vi "test-trapezoid-profile-switch-goal-in-middle-2.vi"() -> ()   [LabVIEW 2019]
uses:
  <vilib>/Rock Robotics/WPI/ThirdParty/JAS_Junk/TrajLib/TRAPEZOID_PROFILE_STATE.ctl
  <vilib>/Rock Robotics/WPI/ThirdParty/JAS_Junk/TrajLib/TRAPEZOID_PROFILE.ctl
  <vilib>/Rock Robotics/WPI/ThirdParty/JAS_Junk/TrajLib/TRAPEZOID_PROFILE_CONSTRAINT.ctl
  <vilib>/Rock Robotics/WPI/ThirdParty/JAS_Junk/TrajLib/TrapProfile_ShouldFlipAcceleration.vi
  <vilib>/Rock Robotics/WPI/ThirdParty/JAS_Junk/TrajLib/TrapProfile_Direct.vi
  <vilib>/Rock Robotics/SystemInterfaces/NetworkCommunication/NetComm_UsageReport_report.vi
  <vilib>/Rock Robotics/WPI/ThirdParty/JAS_Junk/TrajLib/Util_LibraryGlobals.vi
  <vilib>/Rock Robotics/WPI/ThirdParty/JAS_Junk/TrajLib/Trajectory_Library.lvlib
panel:
  out "TRAPEZOID_PROFILE":T1 {"Goal"."Velocity" format="%16_6e"; "Goal"."Position" format="%16_6e"; "Initial"."Velocity" format="%16_6e"; "Initial"."Position" format="%16_6e"; "Constraints"."MaxAcceleration" format="%16_6e"; "Constraints"."MaxVelocity" format="%16_6e"; "EndDecel" format="%16_6e"; "EndFullSpeed" format="%16_6e"; "EndAccel" format="%16_6e"}
  out "State":T3 {"Velocity" format="%16_6e"; "Position" format="%16_6e"}
  out "Waveform Chart":T4(graph)
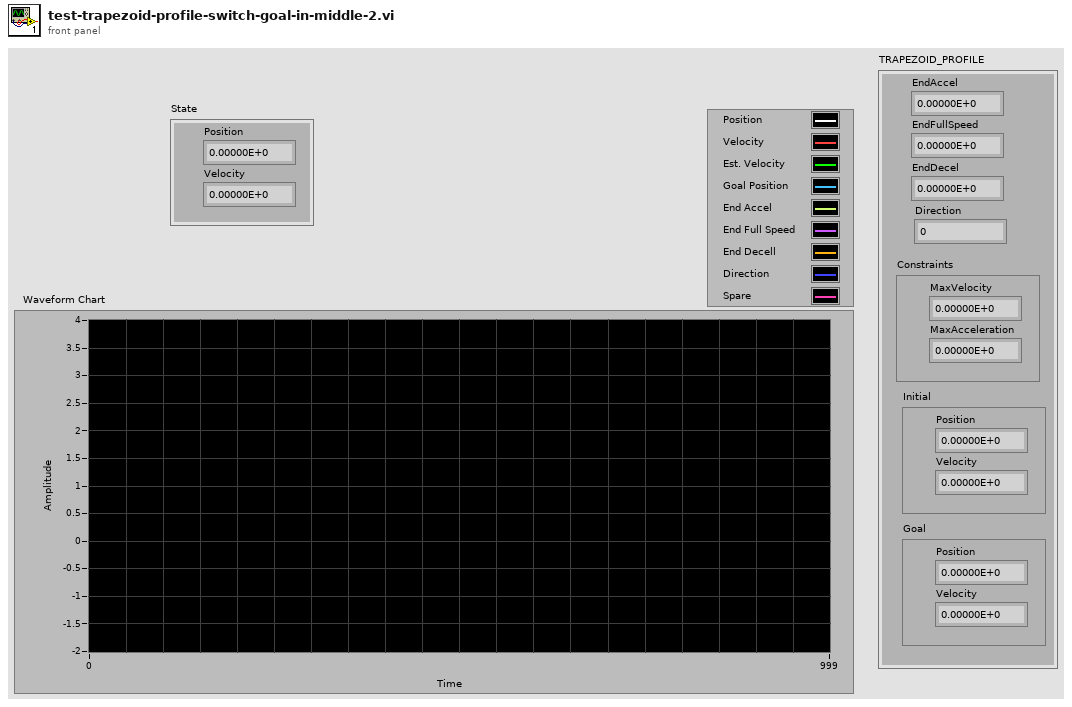
[diagram p1: front panel]
types:
  T1 = typedef "Trajectory_Library.lvlib/TRAPEZOID_PROFILE.ctl" = cluster{"EndAccel":dbl, "EndFullSpeed":dbl, "EndDecel":dbl, "Direction":i32, "Constraints":T2, "Initial":T3, "Goal":T3}
  T2 = typedef "Trajectory_Library.lvlib/TRAPEZOID_PROFILE_CONSTRAINT.ctl" = cluster{"MaxVelocity":dbl, "MaxAcceleration":dbl}
  T3 = typedef "Trajectory_Library.lvlib/TRAPEZOID_PROFILE_STATE.ctl" = cluster{"Position":dbl, "Velocity":dbl}
  T4 = cluster{"Position":dbl, "Velocity":dbl, dbl, "Position":dbl, "EndAccel":dbl, "EndFullSpeed":dbl, "EndDecel":dbl, "Direction":i32, "Position":dbl}
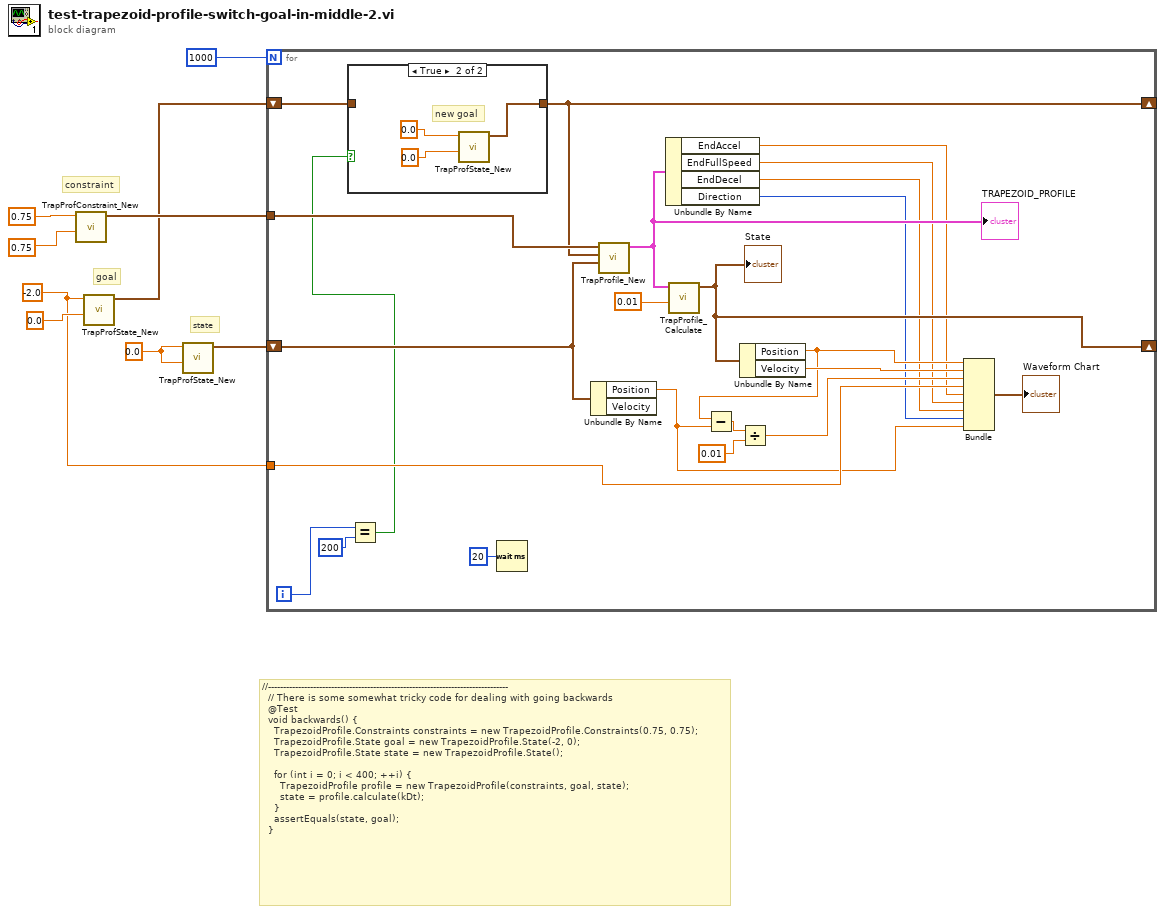
[diagram p0: block diagram]
diagram:
  w5 = 0.0 ("Position")
  w2 = -2.0 ("Position")
  # "state"
  # "//--------------------------------------------------------------------------------\n  // There is some somewhat tricky code for dealing with going backwards\n  @Test\n  void backwards() {\n    TrapezoidProfile.Constraints constraints = new TrapezoidProfile.Constraints(0.75, 0.75);\n    TrapezoidProfile.State goal = new TrapezoidProfile.State(-2, 0);\n    TrapezoidProfile.State state = new TrapezoidProfile.State();\n\n    for (int i = 0; i < 400; ++i) {\n      TrapezoidProfile profile = new TrapezoidProfile(constraints, goal, state);\n      state = profile.calculate(kDt);\n    }\n    assertEquals(state, goal);\n  }"
  # "goal"
  # "constraint"
  n1 = call <vilib>:"TrapProfConstraint_New.vi"("Max Accel"=0.75, "Max Speed (M/S)"=0.75) -> ("TRAPEZOID_PROFILE_CONSTRAINT"=w3:T2)  [unwired: 9 in]
  n2 = call <vilib>:"TrapProfState_New.vi"("Velocity"=0.0, "Position"=w2) -> ("TRAPEZOID_PROFILE_STATE"=w1:T3)  [unwired: 9 in]
  n3 = call <vilib>:"TrapProfState_New.vi"("Velocity"=w5, "Position"=w5) -> ("TRAPEZOID_PROFILE_STATE"=w4:T3)  [unwired: 9 in]
  n4 = for {
    N: 1000 -> [_]
    shift-right: [w23] -> _
    shift-left: w4 -> [w28]
    tunnel: w2 -> [w22]
    tunnel: w3 -> [w15]
    shift-right: [w10] -> _
    shift-left: w1 -> [w14]
    i -> [w13]
    n5 = Equal?(x=w13, y=200) -> (x = y?=w11:bool)
    n6 = case shown="True" w11 {
      tunnel: w14 -> [w33 _]
      tunnel: [w33 w34] -> w10
      frame False {
      }
      frame True {
        # "new goal"
        n7 = call <vilib>:"TrapProfState_New.vi"("Velocity"=0.0, "Position"=0.0) -> ("TRAPEZOID_PROFILE_STATE"=w34:T3)  [unwired: 9 in]
      }
    }
    n8 = Wait (ms)(milliseconds to wait=u32 20) -> ()  [unwired: 1 out]
    n9 = Unbundle By Name(w28) -> ("Position"=w16:dbl)  [unwired: 1 out]
    n10 = call <vilib>:"TrapProfile_New.vi"("Initial"=w28, "Goal"=w10, "Constraints"=w15) -> ("TRAPEZOID_PROFILE"=w21:T1)  [unwired: 8 in]
    "TRAPEZOID_PROFILE" <- w21
    n11 = Unbundle By Name(w21) -> ("EndAccel"=w20:dbl, "EndFullSpeed"=w19:dbl, "EndDecel"=w18:dbl, "Direction"=w17:i32)
    n12 = call <vilib>:"TrapProfile_Calculate.vi"("Time"=0.01, "TRAPEZOID_PROFILE"=w21) -> ("State"=w23:T3)  [unwired: 9 in]
    "State" <- w23
    n13 = Unbundle By Name(w23) -> ("Position"=w27:dbl, "Velocity"=w30:dbl)
    n14 = Subtract(x=w27, y=w16) -> (x-y=w26:dbl)
    n15 = Divide(x=w26, y=0.01) -> (x/y=w24:dbl)
    n16 = Bundle("Position"=w27, "Velocity"=w30, w24, "Position"=w22, "EndAccel"=w20, "EndFullSpeed"=w19, "EndDecel"=w18, "Direction"=w17, "Position"=w16) -> (→"Waveform Chart":T4)  [unwired: 1 in]
  }
